vi "Decode ABORT Message.vi"(8 "error in (no error)":errorcluster, 11 "Data":variant) -> (2 "Sender":string, 3 "Abort":bool)   [LabVIEW 2026, in "TALOS.lvlib" / "Guardian.lvlib" / "Guardian.lvclass"]
uses:
  Guardian.lvclass
  TALOS.lvlib
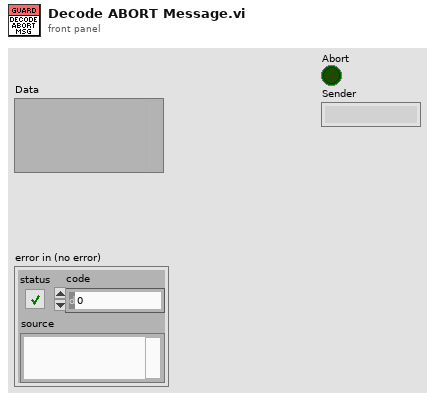
[diagram p1: front panel]
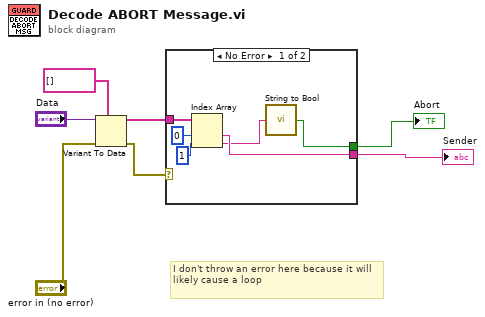
[diagram p0: block diagram]
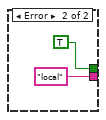
[diagram p2: hidden frame]
diagram:
  # "I don't throw an error here because it will likely cause a loop"
  n1 = Variant To Data(error in="error in (no error)", type=string[] [], Variant="Data") -> (data=w1:string[], error out=w5:errorcluster)
  n2 = case shown="No Error" w5 {
    tunnel: w1 -> [w13 _]
    tunnel: [w10 "local" ("Sender")] -> w3
    tunnel: [w8 TRUE ("New Abort Value")] -> w4
    frame No Error {
      n3 = Index Array(array=w13, index #1=0 ("index"), index #2=1 ("index")) -> (element #1=w10:string, element #2=w9:string)
      n4 = call "String to Bool.vi"("String"=w9) -> ("Boolean"=w8:bool)
    }
    frame Error {
    }
  }
  "Abort" <- w4
  "Sender" <- w3
